vi "ABR3-Init Data File.vi"(0 "Stimulus":T3={"Ear"=enum."Left", "Waveform"=enum."FILE", "Frequency (kHz)"="", "Rep rate (/sec)"=80.0, "Alternate Polarity"=FALSE, "WavFiles"="", "Level (dB SPL)"=30.0, "WavFolder"=path "", "Info"=""}, 1 "Experiment Info":T1, 5 "CAP or ABR":u16(ring)=1 items=["CAP", "ABR"], 7 "Response":T2={"Gain"=10000, "Averages"=512, "Window (ms)"=8.5, "Thr Fast Steps"=8.5} {"Thr Fast Steps" format="%.2f"; "Window (ms)" format="%.2f"}, 9 "Rep Rate (Hz)":dbl=10.0, 11 "error in (no error)":errorcluster, 12 "Freq (kHz)":dbl, 13 "Sample Interval (µsec)":dbl=10.0) -> (3 "State (out)":T1, 6 "Datafile path":path, 15 "error out":errorcluster)   [LabVIEW 2020]
uses:
  Utility VIs/Type Defs/Left-Right ring.ctl
  TypeDefs/ABR Response.ctl
  CFTS Main Panel SubVIs/CFTS-Experiment State.ctl
  TypeDefs/ABR3-Stimulus.ctl
  TypeDefs/ABR-Waveform Enum.ctl
panel:
  in  "Acoustic System":u16(ring)=2 items=["", "ER-10c System", "RS Tweeter", "Starship System"]
  in  "NOTES":string
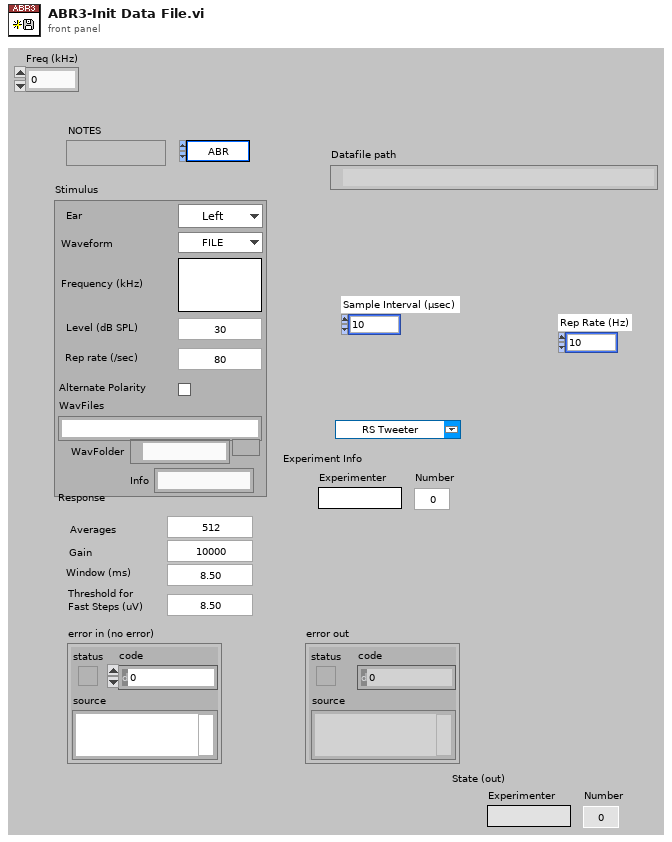
[diagram p1: front panel]
types:
  T1 = typedef "CFTS-Experiment State.ctl" = cluster{"Experimenter":string, "Number":u32, "Right":string, "Left":string, "Data Folder":path, "State File":path, "Version Info":string, "End Exposure Time":dbl, "Exposure Duration":string, "Run #":cluster{"CAP":i16, "ABR":i16, "DP":i16, "VsEP":i16, "MeasSeq":i16, "SubSeq":i16, "SFOAE":i16}}
  T2 = typedef "ABR Response.ctl" = cluster{"Gain":i32, "Averages":i32, "Window (ms)":sgl, "Thr Fast Steps":sgl}
  T3 = typedef "ABR3-Stimulus.ctl" = cluster{"Ear":T4, "Waveform":T5, "Frequency (kHz)":string, "Rep rate (/sec)":dbl, "Alternate Polarity":bool, "WavFiles":string, "Level (dB SPL)":dbl, "WavFolder":path, "Info":string}
  T4 = typedef "Left-Right ring.ctl" = enum16{"Right", "Left"}
  T5 = typedef "ABR-Waveform Enum.ctl" = enum16{"TONE PIP", "CLICK", "FILE", "CHIRP", "NOISE", "VERHULST"}
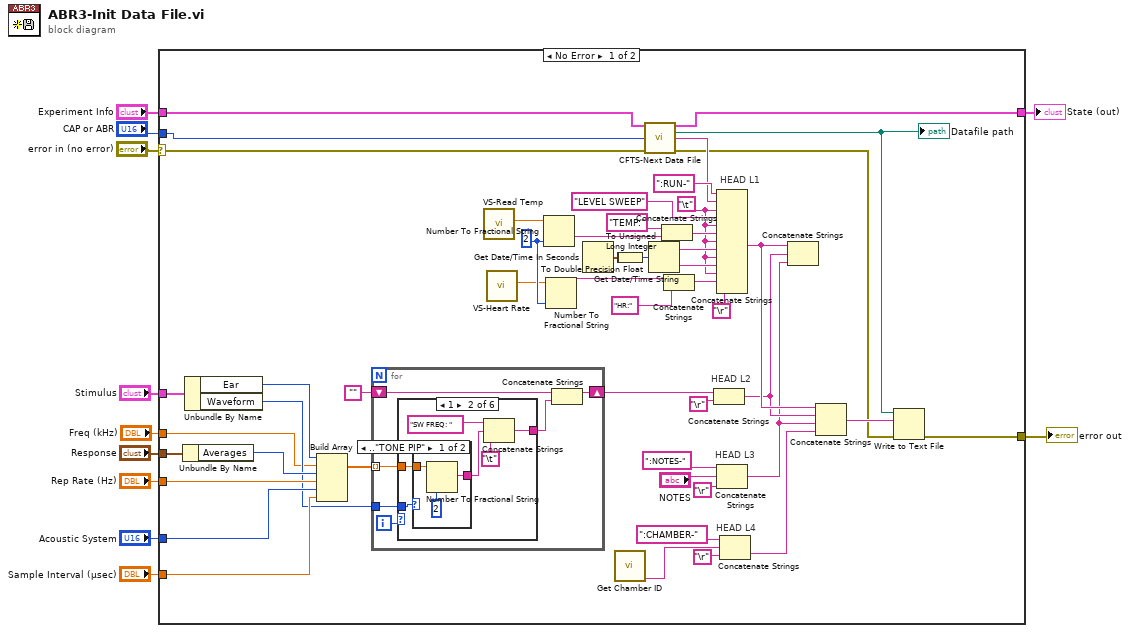
[diagram p0: block diagram]
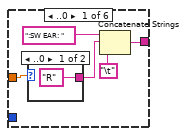
[diagram p2: hidden frame]
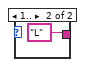
[diagram p3: hidden frame]
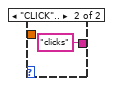
[diagram p4: hidden frame]
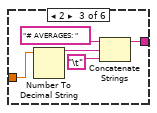
[diagram p5: hidden frame]
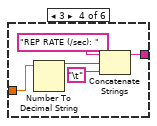
[diagram p6: hidden frame]
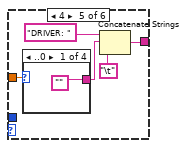
[diagram p7: hidden frame]
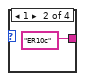
[diagram p8: hidden frame]
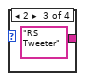
[diagram p9: hidden frame]
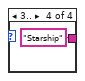
[diagram p10: hidden frame]
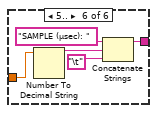
[diagram p11: hidden frame]
diagram:
  n1 = case shown="No Error" "error in (no error)" {
    selector: "error in (no error)" -> [w18 w110]
    tunnel: "Sample Interval (µsec)" -> [w32 _]
    tunnel: "Acoustic System" -> [w31 _]
    tunnel: "Rep Rate (Hz)" -> [w25 _]
    tunnel: "Stimulus" -> [w24 _]
    tunnel: "Response" -> [w21 _]
    tunnel: [w19 w110] -> w6
    tunnel: "CAP or ABR" -> [w17 _]
    tunnel: "Experiment Info" -> [w16 w109]
    tunnel: [w14 w109] -> w2
    tunnel: "Freq (kHz)" -> [w12 _]
    frame No Error {
      w40 = "\t"
      w37 = 2
      # "HEAD L4"
      # "HEAD L1"
      # "HEAD L2"
      # "HEAD L3"
      n2 = Unbundle By Name(w21) -> ("Averages"=w48:i32)
      n3 = Unbundle By Name(w24) -> ("Ear"=w23:T4, "Waveform"=w22:T5)
      n4 = Build Array(w23, w12, w48, w25, w31, w32) -> (w43:dbl[])
      n5 = for {
        shift-right: [w64] -> w58
        shift-left: "" -> [w66]
        tunnel: w22 -> [w62]
        tunnel: w43 -> [w63] mode=indexing
        i -> [w67]
        n6 = case shown="1" w67 {
          tunnel: w62 -> [_ w77 _ _ _ _]
          tunnel: w63 -> [w69 w76 w85 w90 w96 w104]
          tunnel: [w71 w79 w86 w91 w98 w105] -> w65
          frame ..0 {
            n7 = case shown="..0" w69 {
              tunnel: ["R" "L"] -> w68
              frame ..0 {
              }
              frame 1.. {
              }
            }
            n8 = Concatenate Strings(":SW EAR: ", w68, "\t") -> (w71:string)
          }
          frame 1 {
            n9 = case shown="..\"TONE PIP\"" w77 {
              tunnel: [w82 "clicks"] -> w75
              tunnel: w76 -> [w83 _]
              frame .."TONE PIP" {
                n10 = Number To Fractional String(number=w83, precision (6)=2) -> (F-format string=w82:string)  [unwired: 2 in]
              }
              frame "CLICK".. {
              }
            }
            n11 = Concatenate Strings("SW FREQ: ", w75, "\t") -> (w79:string)
          }
          frame 2 {
            n12 = Number To Decimal String(number=w85) -> (decimal integer string=w88:string)  [unwired: 1 in]
            n13 = Concatenate Strings("# AVERAGES: ", w88, "\t") -> (w86:string)
          }
          frame 3 {
            n14 = Number To Decimal String(number=w90) -> (decimal integer string=w93:string)  [unwired: 1 in]
            n15 = Concatenate Strings("REP RATE (/sec): ", w93, "\t") -> (w91:string)
          }
          frame 4 {
            n16 = case shown="..0" w96 {
              tunnel: ["" "ER10c" "RS Tweeter" "Starship"] -> w95
              frame ..0 {
              }
              frame 1 {
              }
              frame 2 {
              }
              frame 3.. {
              }
            }
            n17 = Concatenate Strings("DRIVER: ", w95, "\t") -> (w98:string)
          }
          frame 5.. {
            n18 = Number To Decimal String(number=w104) -> (decimal integer string=w107:string)  [unwired: 1 in]
            n19 = Concatenate Strings("SAMPLE (µsec): ", w107, "\t") -> (w105:string)
          }
        }
        n20 = Concatenate Strings(w66, w65) -> (w64:string)
      }
      n21 = call "VS-Read Temp.vi"() -> ("Temp (C)"=w27:dbl)  [unwired: 10 in, 1 out]
      n22 = call "VS-Heart Rate.vi"() -> ("Heart Rate (bpm)"=w26:dbl)  [unwired: 11 in]
      n23 = Number To Fractional String(number=w27, precision (6)=w37) -> (F-format string=w55:string)  [unwired: 2 in]
      n24 = Number To Fractional String(number=w26, precision (6)=w37) -> (F-format string=w36:string)  [unwired: 2 in]
      n25 = Get Date/Time In Seconds() -> (seconds since 1Jan1904=w29:timestamp)
      n26 = To Double Precision Float(number=w29) -> (double precision float=w30:dbl)
      n27 = To Unsigned Long Integer(number=w30) -> (unsigned 32bit integer=w61:u32)
      n28 = call "Get Chamber ID.vi"() -> ("Chamber name"=w13:string)  [unwired: 4 in, 2 out]
      n29 = call "CFTS-Next Data File.vi"("Expt State"=w16, "Data Type"=w17, "error in (no error)"=w18) -> ("Expt State out"=w14:T1, "Datafile path"=w15:path, "run #"=w28:string, "error out"=w20:errorcluster)  [unwired: 8 in, 1 out]
      "Datafile path" <- w15
      n30 = Get Date/Time String(seconds (now)=w61) -> (date string=w46:string, time string=w45:string)  [unwired: 2 in]
      n31 = Concatenate Strings("TEMP:", w55) -> (w47:string)
      n32 = Concatenate Strings(w36, "HR:") -> (w39:string)
      n33 = Concatenate Strings(w58, "\r") -> (w53:string)
      n34 = Concatenate Strings(":RUN-", w28, w40, "LEVEL SWEEP", w40, w47, w40, w46, w40, w45, w40, w39, "\r") -> (w54:string)
      n35 = Concatenate Strings(":NOTES-", "NOTES", "\r") -> (w50:string)
      n36 = Concatenate Strings(":CHAMBER-", w13, "\r") -> (w33:string)
      n37 = Concatenate Strings(w54, w53, w50) -> ()  [unwired: 1 out]
      n38 = Concatenate Strings(w54, w53, w50, w33) -> (w42:string)
      n39 = Write to Text File(file (use dialog)=w15, text=w42, error in=w20) -> (error out=w19:errorcluster)  [unwired: 1 in, 2 out]
    }
    frame Error {
    }
  }
  "error out" <- w6
  "State (out)" <- w2
